vi "FPGAStartRun.vi"(11 "targetVIref":T1) -> (3 "done":bool)   [LabVIEW 2020, in "NI_TargetHelper.lvlib"]
uses:
  <vilib>/TargetSupport/NI_TargetHelper/NI_TargetHelper.lvlib
  <vilib>/TargetSupport/NI_TargetHelper/Instance VIref.ctl
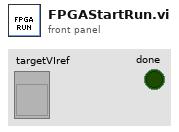
[diagram p1: front panel]
types:
  T1 = typedef "NI_TargetHelper.lvlib/Instance VIref.ctl" = refnum<vi>
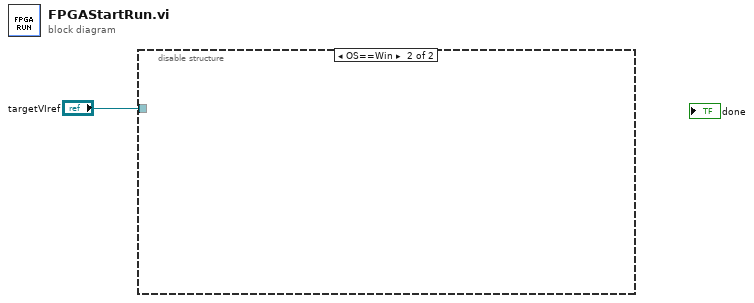
[diagram p0: block diagram]
diagram:
  n1 = disable-structure shown="OS==Win" {
    disable-tunnel: "targetVIref" -> [_ _]
    frame condition #0 (active) {
    }
    frame condition #1 {
    }
  }
